vi "Build DB Creation String.vi"(8 "Error In":errorcluster) -> (0 "Error Out":errorcluster, 3 "DB Creation String":string)   [LabVIEW 2023]
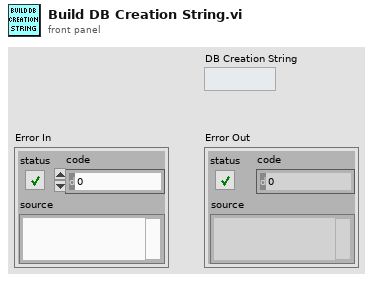
[diagram p1: front panel]
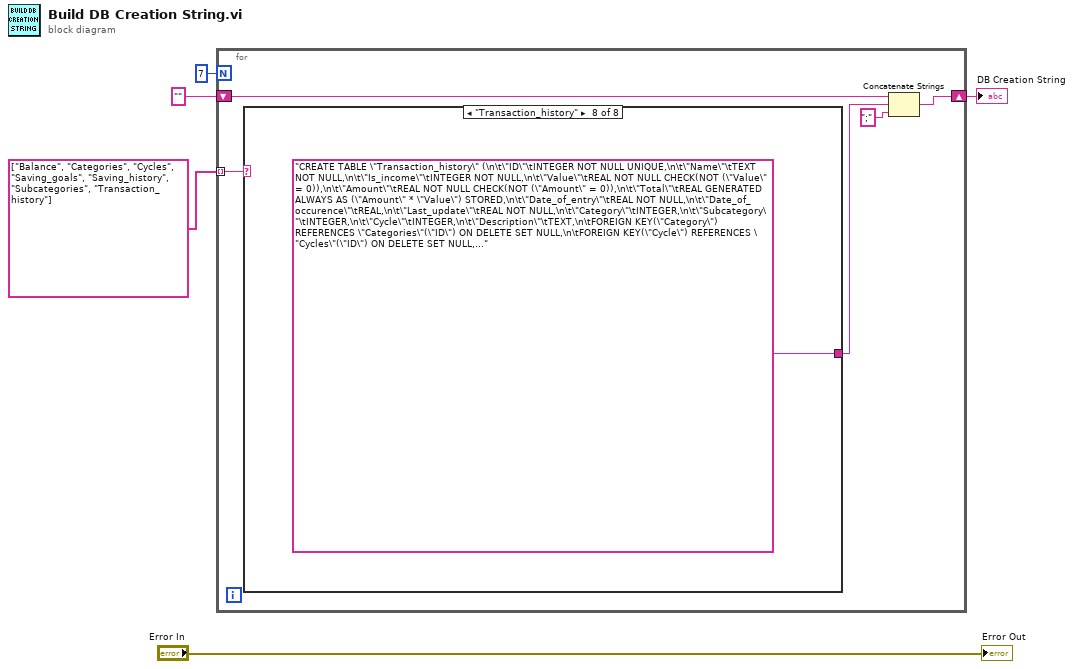
[diagram p0: block diagram]
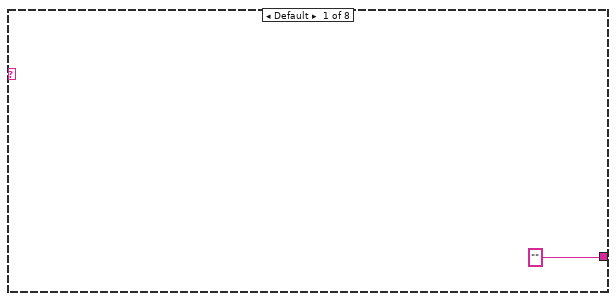
[diagram p2: hidden frame]
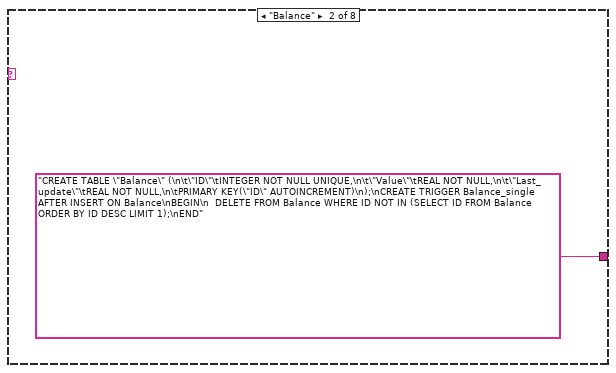
[diagram p3: hidden frame]
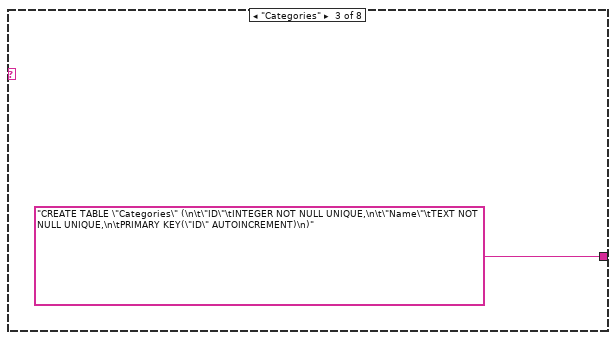
[diagram p4: hidden frame]
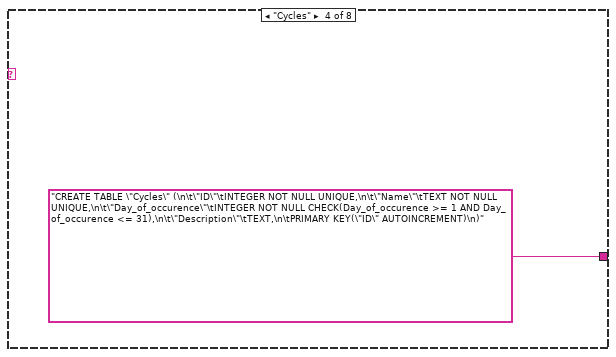
[diagram p5: hidden frame]
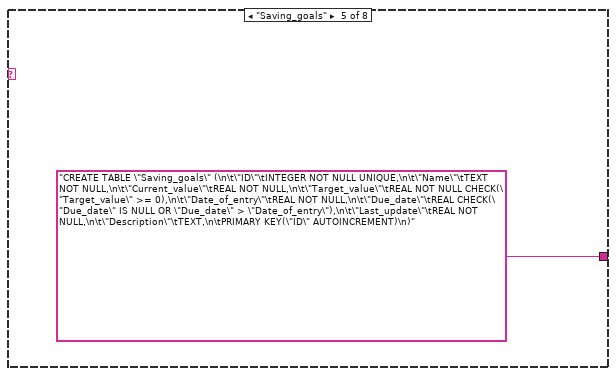
[diagram p6: hidden frame]
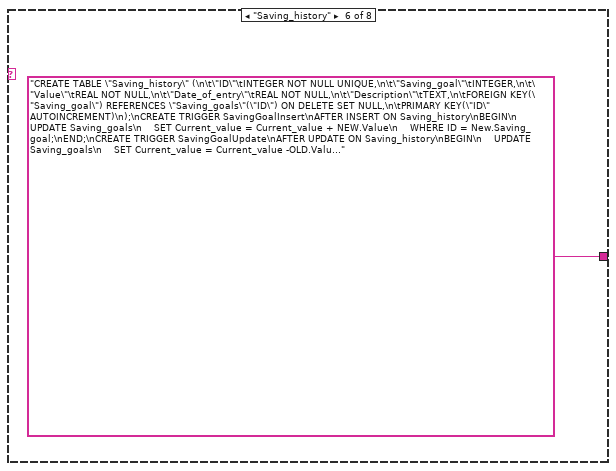
[diagram p7: hidden frame]
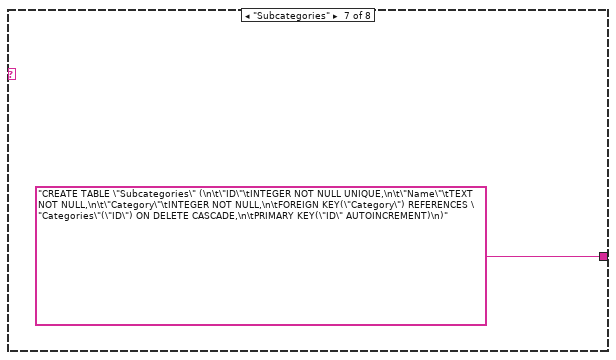
[diagram p8: hidden frame]
diagram:
  n1 = for {
    N: 7 -> [_]
    shift-right: [w9] -> w4
    shift-left: "" -> [w6]
    tunnel: string[] ["Balance", "Categories", "Cycles", "Saving_goals", "Saving_history", "Subcategories", "Transaction_history"] -> [w8] mode=indexing
    n2 = case shown="\"Transaction_history\"" w8 {
      tunnel: ["" "CREATE TABLE \"Balance\" (\n\t\"ID\"\tINTEGER NOT NULL UNIQUE,\n\t\"Value\"\tREAL NOT NULL,\n\t\"Last_update\"\tREAL NOT NULL,\n\tPRIMARY KEY(\"ID\" AUTOINCREMENT)\n);\nCREATE TRIGGER Balance_single AFTER INSERT ON Balance\nBEGIN\n  DELETE FROM Balance WHERE ID NOT IN (SELECT ID FROM Balance ORDER BY ID DESC LIMIT 1);\nEND" "CREATE TABLE \"Categories\" (\n\t\"ID\"\tINTEGER NOT NULL UNIQUE,\n\t\"Name\"\tTEXT NOT NULL UNIQUE,\n\tPRIMARY KEY(\"ID\" AUTOINCREMENT)\n)" "CREATE TABLE \"Cycles\" (\n\t\"ID\"\tINTEGER NOT NULL UNIQUE,\n\t\"Name\"\tTEXT NOT NULL UNIQUE,\n\t\"Day_of_occurence\"\tINTEGER NOT NULL CHECK(Day_of_occurence >= 1 AND Day_of_occurence <= 31),\n\t\"Description\"\tTEXT,\n\tPRIMARY KEY(\"ID\" AUTOINCREMENT)\n)" "CREATE TABLE \"Saving_goals\" (\n\t\"ID\"\tINTEGER NOT NULL UNIQUE,\n\t\"Name\"\tTEXT NOT NULL,\n\t\"Current_value\"\tREAL NOT NULL,\n\t\"Target_value\"\tREAL NOT NULL CHECK(\"Target_value\" >= 0),\n\t\"Date_of_entry\"\tREAL NOT NULL,\n\t\"Due_date\"\tREAL CHECK(\"Due_date\" IS NULL OR \"Due_date\" > \"Date_of_entry\"),\n\t\"Last_update\"\tREAL NOT NULL,\n\t\"Description\"\tTEXT,\n\tPRIMARY KEY(\"ID\" AUTOINCREMENT)\n)" "CREATE TABLE \"Saving_history\" (\n\t\"ID\"\tINTEGER NOT NULL UNIQUE,\n\t\"Saving_goal\"\tINTEGER,\n\t\"Value\"\tREAL NOT NULL,\n\t\"Date_of_entry\"\tREAL NOT NULL,\n\t\"Description\"\tTEXT,\n\tFOREIGN KEY(\"Saving_goal\") REFERENCES \"Saving_goals\"(\"ID\") ON DELETE SET NULL,\n\tPRIMARY KEY(\"ID\" AUTOINCREMENT)\n);\nCREATE TRIGGER SavingGoalInsert\nAFTER INSERT ON Saving_history\nBEGIN\n    UPDATE Saving_goals\n    SET Current_value = Current_value + NEW.Value\n    WHERE ID = New.Saving_goal;\nEND;\nCREATE TRIGGER SavingGoalUpdate\nAFTER UPDATE ON Saving_history\nBEGIN\n    UPDATE Saving_goals\n    SET Current_value = Current_value -OLD.Value+ NEW.Value\n    WHERE ID = New.Saving_goal;\nEND" "CREATE TABLE \"Subcategories\" (\n\t\"ID\"\tINTEGER NOT NULL UNIQUE,\n\t\"Name\"\tTEXT NOT NULL,\n\t\"Category\"\tINTEGER NOT NULL,\n\tFOREIGN KEY(\"Category\") REFERENCES \"Categories\"(\"ID\") ON DELETE CASCADE,\n\tPRIMARY KEY(\"ID\" AUTOINCREMENT)\n)" "CREATE TABLE \"Transaction_history\" (\n\t\"ID\"\tINTEGER NOT NULL UNIQUE,\n\t\"Name\"\tTEXT NOT NULL,\n\t\"Is_income\"\tINTEGER NOT NULL,\n\t\"Value\"\tREAL NOT NULL CHECK(NOT (\"Value\" = 0)),\n\t\"Amount\"\tREAL NOT NULL CHECK(NOT (\"Amount\" = 0)),\n\t\"Total\"\tREAL GENERATED ALWAYS AS (\"Amount\" * \"Value\") STORED,\n\t\"Date_of_entry\"\tREAL NOT NULL,\n\t\"Date_of_occurence\"\tREAL,\n\t\"Last_update\"\tREAL NOT NULL,\n\t\"Category\"\tINTEGER,\n\t\"Subcategory\"\tINTEGER,\n\t\"Cycle\"\tINTEGER,\n\t\"Description\"\tTEXT,\n\tFOREIGN KEY(\"Category\") REFERENCES \"Categories\"(\"ID\") ON DELETE SET NULL,\n\tFOREIGN KEY(\"Cycle\") REFERENCES \"Cycles\"(\"ID\") ON DELETE SET NULL,\n\tFOREIGN KEY(\"Subcategory\") REFERENCES \"Subcategories\"(\"ID\") ON DELETE SET NULL,\n\tPRIMARY KEY(\"ID\" AUTOINCREMENT));\nCREATE TRIGGER ReplaceNullValueInsert\nAFTER INSERT ON Transaction_history\nBEGIN\n    UPDATE Transaction_history\n    SET Date_of_occurence = COALESCE(Date_of_occurence, Date_of_entry)\n    WHERE ID = NEW.ID;\nEND;\nCREATE TRIGGER ReplaceNullValueUpdate\nAFTER UPDATE OF Date_of_occurence ON Transaction_history\nBEGIN\n    UPDATE Transaction_history\n    SET Date_of_occurence = COALESCE(Date_of_occurence, Date_of_entry)\n    WHERE ID = NEW.ID;\nEND;"] -> w7
      frame Default {
      }
      frame "Balance" {
      }
      frame "Categories" {
      }
      frame "Cycles" {
      }
      frame "Saving_goals" {
      }
      frame "Saving_history" {
      }
      frame "Subcategories" {
      }
      frame "Transaction_history" {
      }
    }
    n3 = Concatenate Strings(w6, w7, ";" ("string")) -> (w9:string)
  }
  "DB Creation String" <- w4
  "Error Out" <- "Error In"
